vi "Math - Signals Statistics.vi"(0 "reference in":refnum<class "GSwFormDSP.lvclass">, 5 "error in (no error)":errorcluster) -> (7 "RMS":dbl[](array[numeric]), 9 "Min's":dbl[](array[numeric]), 11 "Max's":dbl[](array[numeric]), 13 "Mean/DC":dbl[](array[numeric]), 14 "reference in":refnum<class "GSwFormDSP.lvclass">, 17 "Nb Samples":i32[](array[numeric]), 18 "Durations (msec)":dbl[](array[numeric]), 19 "error out":errorcluster)   [LabVIEW 2022 SP3, in "GSwFormDSP.lvclass"]
uses:
  GSwFormDSP.lvclass
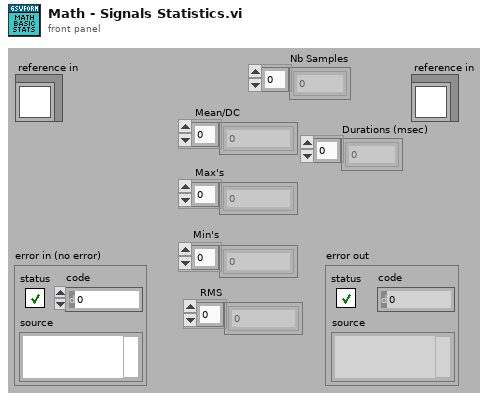
[diagram p1: front panel]
types:
  T1 = typedef "GSwFormDSP.lvclass/ObjectAttributes.ctl" = cluster{"Wform Ref":refnum<data-value>, "Nb Signals":i32, "Spectral Function Parameters":T2, "FFT":waveform(cdb)[], "Nb FFT":i32, "Nb Averages":i32[], "Reference Indexes":i32[], "Response Indexes":i32[], "Coherence":waveform(dbl)[], "TDF Parameters":T4, "DAQ":cluster{"Duration (sec)":dbl, "Buffer Size (Samples)":i32, "Offset (Samples)":i32}, "Filter Impulse Response (TDF)":waveform(dbl), "Sound Playback":T5}
  T2 = typedef "GSwFormDSP.lvclass/Spectral Parameters.ctl" = cluster{"Frequency resolution (Hz)":dbl, "Overlap":dbl, "Window":T3}
  T3 = typedef "NI_AALPro.lvlib/windowTd.ctl" = u32
  T4 = typedef "GSwFormDSP.lvclass/TDF Parameters.ctl" = cluster{"Filter":enum32{"Lowpass", "Highpass", "Bandpass", "Bandstop"}, "Type:":enum16{"Butterworth", "Chebyshev", "Inv Chebyshev", "Elliptic", "Bessel"}, "LP cutoff freq":dbl, "HP cutoff freq":dbl, "Order":i32, "passband ripple (dB)":dbl, "stopband attenuation (dB)":dbl, "Phaseless Filter":bool, "Include Fade IN and OUT":bool}
  T5 = typedef "GSwFormDSP.lvclass/Sound Playback.ctl" = cluster{"Timer start (ms)":u32, "task ID":T6, "Cursor Init Location (s)":dbl, "SC Volume":dbl}
  T6 = typedef "Sound Output Task ID.ctl" = u32
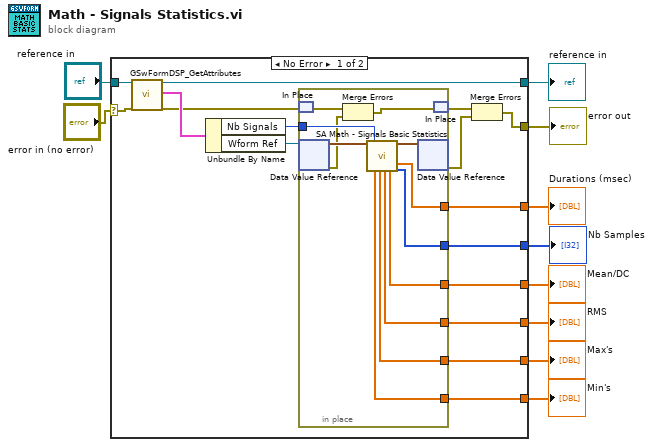
[diagram p0: block diagram]
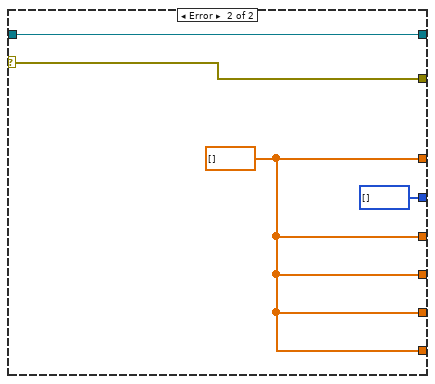
[diagram p2: hidden frame]
diagram:
  n1 = case shown="No Error" "error in (no error)" {
    selector: "error in (no error)" -> [w19 w42]
    tunnel: [w26 w42] -> w9
    tunnel: [w15 w41] -> w7
    tunnel: "reference in" -> [w20 w41]
    tunnel: [w25 w40] -> w6
    tunnel: [w24 w40] -> w5
    tunnel: [w23 w40] -> w4
    tunnel: [w22 w40] -> w3
    tunnel: [w12 i32[] [] ("Nb Samples")] -> w2
    tunnel: [w11 w40] -> w1
    frame No Error {
      n2 = call "GSwFormDSP_GetAttributes.vi"("reference in"=w20, "error in (no error)"=w19) -> ("reference out"=w15:refnum<class "GSwFormDSP.lvclass">, "attributes"=w18:T1, "error out"=w14:errorcluster)  [unwired: 14 in, 1 out]
      n3 = Unbundle By Name(w18) -> ("Nb Signals"=w16:i32, "Wform Ref"=w17:refnum<data-value>)
      n4 = in-place {
        in-place-border: [w36] -> w25
        in-place-border: [w35] -> w24
        in-place-border: [w34] -> w23
        in-place-border: [w33] -> w22
        in-place-border: w16 -> [w32]
        in-place-border: [w28] -> w12
        in-place-border: [w27] -> w11
        n5 = in-place-match #1(w14) -> (w31:errorcluster)
        n6 = in-place-dvr #2(w17) -> (w38:waveform(dbl)[], w30:errorcluster)
        n7 = Merge Errors(w31, w30) -> (w29:errorcluster)
        n8 = call "SA Math - Signals Basic Statistics.vi"("Signal in"=w38, "Nb Signals"=w32) -> ("Min's"=w33:dbl[], "Max's"=w34:dbl[], "RMS"=w35:dbl[], "Mean / DC"=w36:dbl[], "Signal OUT"=w37:waveform(dbl)[], "Durations (msec)"=w27:dbl[], "Nb Samples"=w28:i32[])  [unwired: 11 in]
        n9 = in-place-dvr #2(w37) -> (w21:errorcluster)  [unwired: 1 out]
        n10 = in-place-match #1(w29) -> (w13:errorcluster)
      }
      n11 = Merge Errors(w13, w21) -> (w26:errorcluster)
    }
    frame Error {
      w40 = dbl[] []
    }
  }
  "error out" <- w9
  "reference in" <- w7
  "Mean/DC" <- w6
  "Max's" <- w4
  "Min's" <- w3
  "RMS" <- w5
  "Nb Samples" <- w2
  "Durations (msec)" <- w1
